vi "Error_Handle.vi"(8 "error in (no error)":errorcluster, 11 "queue In":refnum<queue>) -> (0 "error out":errorcluster, 3 "queue Out":refnum<queue>)   [LabVIEW 2014]
uses:
  QSM/TypeDef.ctl
  QSM/Queue_Library.lvlib
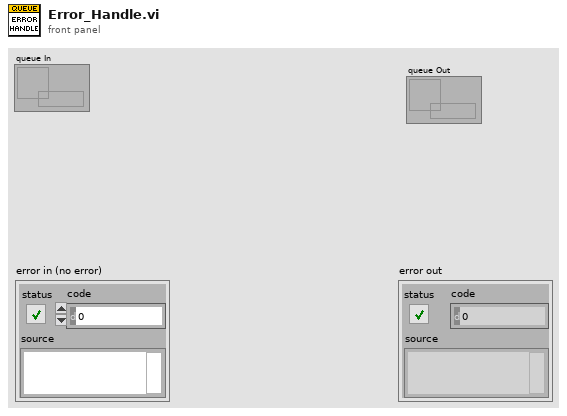
[diagram p1: front panel]
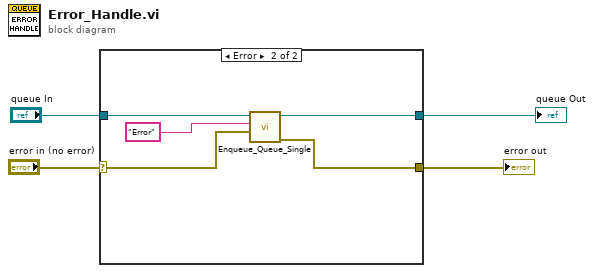
[diagram p0: block diagram]
diagram:
  n1 = case shown="Error" "error in (no error)" {
    selector: "error in (no error)" -> [w5 w7]
    tunnel: "queue In" -> [w6 w11]
    tunnel: [w5 w9] -> w2
    tunnel: [w6 w8] -> w1
    frame No Error {
    }
    frame Error {
      n2 = call "Enqueue_Queue_Single.vi"("Data"=w7, "Command"="Error", "queue In"=w11) -> ("error out"=w9:errorcluster, "queue Out"=w8:refnum<queue>)  [unwired: 7 in]
    }
  }
  "error out" <- w2
  "queue Out" <- w1
